vi "Multiply Matrix.vi"(2 "1st rotation Matrix":dbl[][](array[numeric]) format="%.2f", 3 "2nd rotation Matrix":dbl[][](array[numeric]) format="%.2f") -> (1 "Resultant Matrix":dbl[][](array[numeric]) format="%.2f")   [LabVIEW 2013, in "fick-matrix.lvlib"]
uses:
  fick-matrix.lvlib
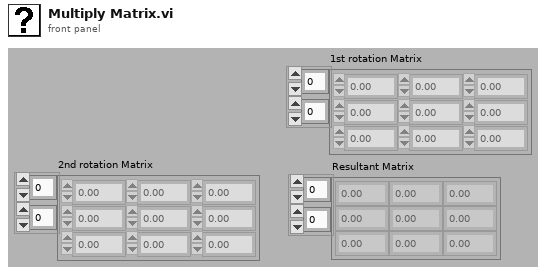
[diagram p1: front panel]
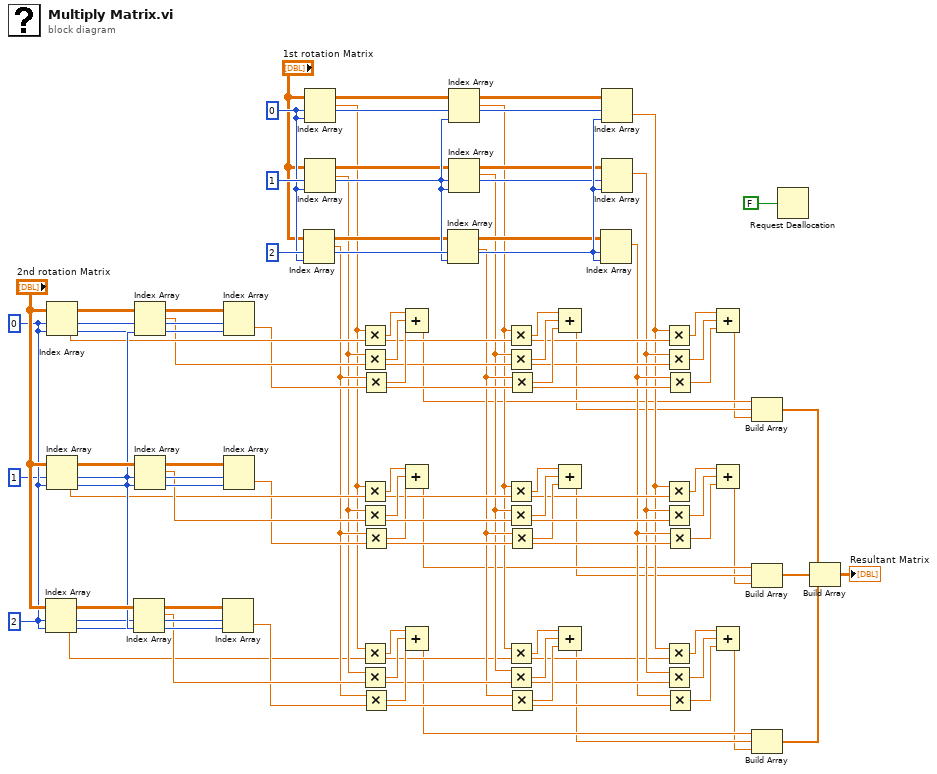
[diagram p0: block diagram]
diagram:
  w61 = 0
  w62 = 1
  w63 = 2
  w64 = 2
  w65 = 1
  w66 = 0
  n1 = Index Array(array="2nd rotation Matrix", index (row)=w64, index (col)=w66) -> (element=w15:dbl)
  n2 = Index Array(array="2nd rotation Matrix", index (row)=w66, index (col)=w66) -> (element=w50:dbl)
  n3 = Index Array(array="2nd rotation Matrix", index (row)=w65, index (col)=w66) -> (element=w37:dbl)
  n4 = Index Array(array="2nd rotation Matrix", index (row)=w64, index (col)=w65) -> (element=w26:dbl)
  n5 = Index Array(array="2nd rotation Matrix", index (row)=w66, index (col)=w65) -> (element=w49:dbl)
  n6 = Index Array(array="2nd rotation Matrix", index (row)=w65, index (col)=w65) -> (element=w47:dbl)
  n7 = Index Array(array="2nd rotation Matrix", index (row)=w64, index (col)=w64) -> (element=w16:dbl)
  n8 = Index Array(array="2nd rotation Matrix", index (row)=w66, index (col)=w64) -> (element=w48:dbl)
  n9 = Index Array(array="2nd rotation Matrix", index (row)=w65, index (col)=w64) -> (element=w36:dbl)
  n10 = Index Array(array="1st rotation Matrix", index (row)=w63, index (col)=w61) -> (element=w25:dbl)
  n11 = Index Array(array="1st rotation Matrix", index (row)=w61, index (col)=w61) -> (element=w23:dbl)
  n12 = Index Array(array="1st rotation Matrix", index (row)=w62, index (col)=w61) -> (element=w24:dbl)
  n13 = Multiply(x=w23, y=w50) -> (x*y=w59:dbl)
  n14 = Multiply(x=w24, y=w49) -> (x*y=w58:dbl)
  n15 = Multiply(x=w23, y=w37) -> (x*y=w38:dbl)
  n16 = Multiply(x=w24, y=w47) -> (x*y=w39:dbl)
  n17 = Multiply(x=w23, y=w15) -> (x*y=w35:dbl)
  n18 = Multiply(x=w24, y=w26) -> (x*y=w34:dbl)
  n19 = Multiply(x=w25, y=w48) -> (x*y=w57:dbl)
  n20 = Multiply(x=w25, y=w36) -> (x*y=w40:dbl)
  n21 = Multiply(x=w25, y=w16) -> (x*y=w33:dbl)
  n22 = Compound Arithmetic op=ADD(w59, w58, w57) -> (w14:dbl)
  n23 = Compound Arithmetic op=ADD(w38, w39, w40) -> (w11:dbl)
  n24 = Compound Arithmetic op=ADD(w35, w34, w33) -> (w8:dbl)
  n25 = Index Array(array="1st rotation Matrix", index (row)=w63, index (col)=w62) -> (element=w22:dbl)
  n26 = Index Array(array="1st rotation Matrix", index (row)=w61, index (col)=w62) -> (element=w20:dbl)
  n27 = Index Array(array="1st rotation Matrix", index (row)=w62, index (col)=w62) -> (element=w21:dbl)
  n28 = Multiply(x=w20, y=w50) -> (x*y=w54:dbl)
  n29 = Multiply(x=w21, y=w49) -> (x*y=w55:dbl)
  n30 = Multiply(x=w20, y=w37) -> (x*y=w43:dbl)
  n31 = Multiply(x=w21, y=w47) -> (x*y=w42:dbl)
  n32 = Multiply(x=w20, y=w15) -> (x*y=w30:dbl)
  n33 = Multiply(x=w21, y=w26) -> (x*y=w31:dbl)
  n34 = Multiply(x=w22, y=w48) -> (x*y=w56:dbl)
  n35 = Multiply(x=w22, y=w36) -> (x*y=w41:dbl)
  n36 = Multiply(x=w22, y=w16) -> (x*y=w32:dbl)
  n37 = Compound Arithmetic op=ADD(w54, w55, w56) -> (w13:dbl)
  n38 = Compound Arithmetic op=ADD(w43, w42, w41) -> (w10:dbl)
  n39 = Compound Arithmetic op=ADD(w30, w31, w32) -> (w7:dbl)
  n40 = Index Array(array="1st rotation Matrix", index (row)=w63, index (col)=w63) -> (element=w19:dbl)
  n41 = Index Array(array="1st rotation Matrix", index (row)=w61, index (col)=w63) -> (element=w17:dbl)
  n42 = Index Array(array="1st rotation Matrix", index (row)=w62, index (col)=w63) -> (element=w18:dbl)
  n43 = Multiply(x=w17, y=w50) -> (x*y=w53:dbl)
  n44 = Multiply(x=w18, y=w49) -> (x*y=w52:dbl)
  n45 = Multiply(x=w17, y=w37) -> (x*y=w44:dbl)
  n46 = Multiply(x=w18, y=w47) -> (x*y=w45:dbl)
  n47 = Multiply(x=w17, y=w15) -> (x*y=w29:dbl)
  n48 = Multiply(x=w18, y=w26) -> (x*y=w28:dbl)
  n49 = Multiply(x=w19, y=w48) -> (x*y=w51:dbl)
  n50 = Multiply(x=w19, y=w36) -> (x*y=w46:dbl)
  n51 = Multiply(x=w19, y=w16) -> (x*y=w27:dbl)
  n52 = Compound Arithmetic op=ADD(w53, w52, w51) -> (w12:dbl)
  n53 = Compound Arithmetic op=ADD(w44, w45, w46) -> (w9:dbl)
  n54 = Compound Arithmetic op=ADD(w29, w28, w27) -> (w6:dbl)
  n55 = Build Array(w14, w13, w12) -> (w5:dbl[])
  n56 = Build Array(w11, w10, w9) -> (w4:dbl[])
  n57 = Build Array(w8, w7, w6) -> (w3:dbl[])
  n58 = Request Deallocation(FALSE ("flag")) -> ()
  n59 = Build Array(w5, w4, w3) -> (→"Resultant Matrix":dbl[][])
